vi "GetOneFrame.vi"(8 "error in (no error)":errorcluster caption="错误输入（无错误）", 9 "nDataSize":u32, 10 "pData":u8[][](array[numeric]), 11 "handle":u64) -> (0 "error out":errorcluster caption="错误输出", 1 "function return":i32, 2 "pData Out":u8[][](array[numeric]), 3 "handle out":u64, 5 "pFrameInfo out":T1)   [LabVIEW 2011, in "MvCameraControl.lvlib"]
doc: "MV_LV_API int __stdcall GetOneFrame( void* handle, unsigned char * pData , unsigned int nDataSize, MV_FRAME_OUT_INFO* pFrameInfo);"
uses:
  MvCameraControl.lvlib
  MvCameraControl.dll
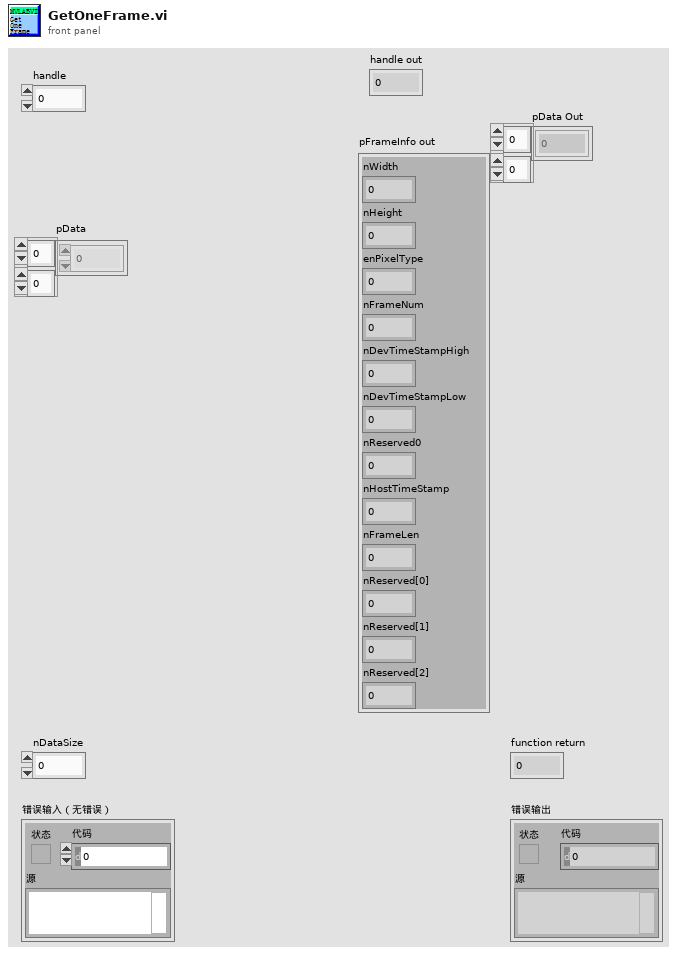
[diagram p1: front panel]
types:
  T1 = cluster{"nWidth":u16, "nHeight":u16, "enPixelType":i32, "nFrameNum":u32, "nDevTimeStampHigh":u32, "nDevTimeStampLow":u32, "nReserved0":u32, "nHostTimeStamp":i64, "nFrameLen":u32, "nReserved[0]":u32, "nReserved[1]":u32, "nReserved[2]":u32}
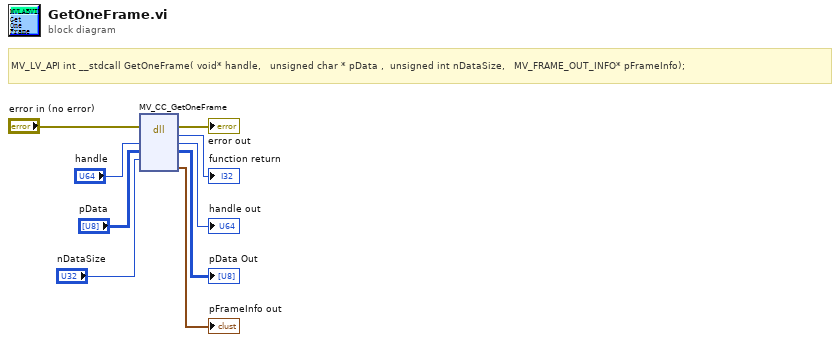
[diagram p0: block diagram]
diagram:
  # "MV_LV_API int __stdcall GetOneFrame( void* handle,   unsigned char * pData ,  unsigned int nDataSize,   MV_FRAME_OUT_INFO* pFrameInfo);"
  n1 = dll-call lib="MvCameraControl.dll" fn="MV_CC_GetOneFrame"(error in="error in (no error)", "handle"="handle", "pData"="pData", "nDataSize"="nDataSize") -> (error out=→"error out":errorcluster, "返回类型"=→"function return":i32, "handle"=→"handle out":u64, "pData"=→"pData Out":u8[][], "pFrameInfo out"=→"pFrameInfo out":T1)  [unwired: 4 in, 1 out]
